vi "Reset.vi"(6 "Settle (1mS)":u32=1, 8 "error in (no error)":errorcluster, 10 "Reset (False: Off)":bool, 11 "VISA resource name":refnum<visa-resource-name>) -> (0 "error out":errorcluster, 3 "VISA resource name out":refnum<visa-resource-name>)   [LabVIEW 2018, in "TDK-Lambda Z.lvlib"]
doc: "Resets the GEN power supply to a known and safe state, if the Reset control is set TRUE (default). This VI will wait for \"Settle\" milliseconds after Reset to allow the output to turn off.\n\nThe reset state includes:\n- Output off\n- Voltage and current program limits to zero\n- Over-voltage protection setting to maximum\n- Under-voltage limit to zero\n- Fold-back protection off\n- Power On (Autostart) is in off state"
uses:
  TDK-Lambda Z.lvlib
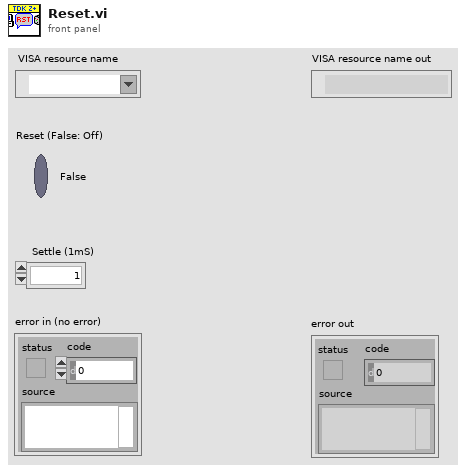
[diagram p1: front panel]
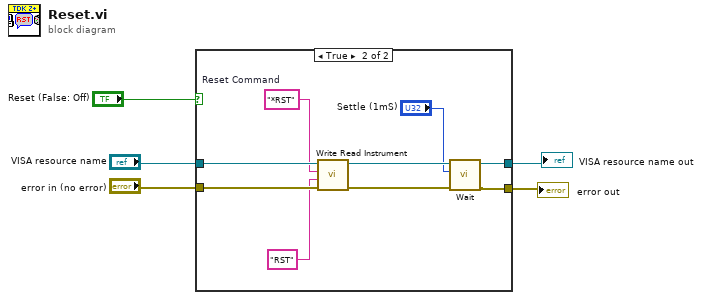
[diagram p0: block diagram]
diagram:
  n1 = case shown="True" "Reset (False: Off)" {
    tunnel: "VISA resource name" -> [w7 w16]
    tunnel: "error in (no error)" -> [w6 w15]
    tunnel: [w7 w12] -> w3
    tunnel: [w6 w11] -> w2
    frame False {
    }
    frame True {
      w9 = "*RST"  # Reset Command
      n2 = call "Write Read Instrument.vi"("error in (no error)"=w15, "GEN  Write Command/Query"="RST" ("Write Command/Query GEN"), "SCPI  Write Command/Query"=w9, "VISA resource name"=w16) -> ("error out"=w13:errorcluster, "VISA resource name out"=w14:refnum<visa-resource-name>)  [unwired: 5 in, 1 out]
      n3 = call "Wait.vi"("error in (no error)"=w13, "Wait (1mS)"="Settle (1mS)", "VISA resource name"=w14) -> ("error out"=w11:errorcluster, "VISA resource name out"=w12:refnum<visa-resource-name>)  [unwired: 7 in]
    }
  }
  "error out" <- w2
  "VISA resource name out" <- w3
